vi "stage to pixel coordinates.vi"(8 "Slide (mm)":T1={"top"=-22300.0, "right"=-13000.0, "width"=60000.0, "height"=60000.0}, 9 "Y in (um)":dbl, 10 "X in (um)":dbl, 11 "image data":T2) -> (1 "Y out (px)":i16, 2 "X out (um)":i16)   [LabVIEW 2018]
uses:
  <vilib>/picture/picture.llb/imagedata.ctl
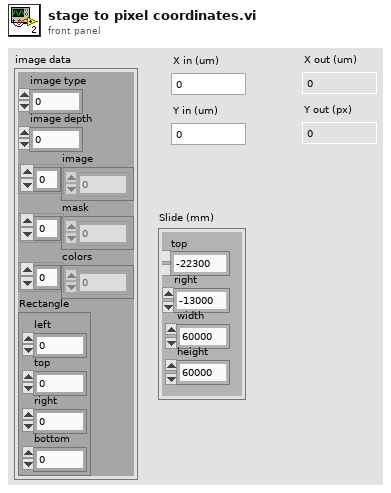
[diagram p1: front panel]
types:
  T1 = cluster{"top":dbl, "right":dbl, "width":dbl, "height":dbl}
  T2 = typedef "imagedata.ctl" = cluster{"image type":i32, "image depth":i32, "image":u8[], "mask":u8[], "colors":u32[], "Rectangle":cluster{"left":i16, "top":i16, "right":i16, "bottom":i16}}
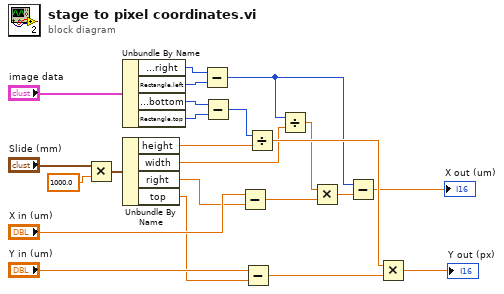
[diagram p0: block diagram]
diagram:
  n1 = Multiply(x="Slide (mm)", y=1000.0) -> (x*y=w5:T1)
  n2 = Unbundle By Name("image data") -> ("Rectangle.right"=w8:i16, "Rectangle.left"=w20:i16, "Rectangle.bottom"=w23:i16, "Rectangle.top"=w22:i16)
  n3 = Unbundle By Name(w5) -> ("height"=w4:dbl, "width"=w3:dbl, "right"=w1:dbl, "top"=w2:dbl)
  n4 = Subtract(x=w8, y=w20) -> (x-y=w15:i16)
  n5 = Subtract(x=w23, y=w22) -> (x-y=w21:i16)
  n6 = Subtract(x="X in (um)", y=w1) -> (x-y=w17:dbl)
  n7 = Subtract(x="Y in (um)", y=w2) -> (x-y=w19:dbl)
  n8 = Divide(x=w21, y=w4) -> (x/y=w18:dbl)
  n9 = Divide(x=w15, y=w3) -> (x/y=w16:dbl)
  n10 = Multiply(x=w16, y=w17) -> (x*y=w14:dbl)
  n11 = Subtract(x=w15, y=w14) -> (x-y=→"X out (um)":dbl)
  n12 = Multiply(x=w18, y=w19) -> (x*y=→"Y out (px)":dbl)
